vi "DataToSend.vi"(8 "error in (no error)":errorcluster, 9 "TimeStamp":timestamp, 10 "Data":string, 11 "Refnum":u64) -> (0 "error out":errorcluster, 3 "DataToSend":refnum<class "DataToSend.lvclass">)   [LabVIEW 2022 SP3, in "TcpServer.lvlib" / "DataToSend.lvclass"]
uses:
  DataToSend.lvclass
  DataToSend.lvclass/DataToSend.ctl
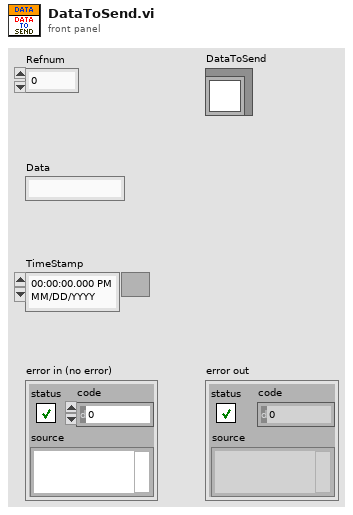
[diagram p1: front panel]
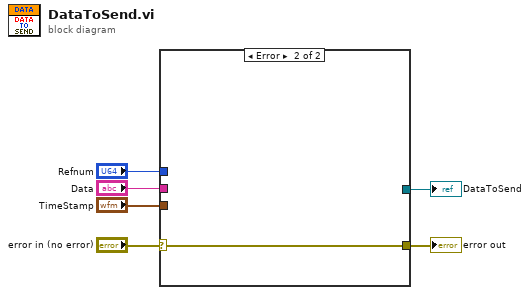
[diagram p0: block diagram]
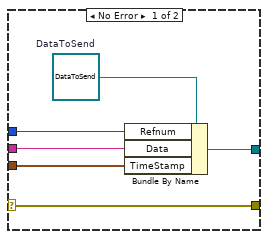
[diagram p2: hidden frame]
diagram:
  n1 = case shown="Error" "error in (no error)" {
    selector: "error in (no error)" -> [w12 w13]
    tunnel: [w12 w13] -> w5
    tunnel: [w10 _] -> w4
    tunnel: "TimeStamp" -> [w9 _]
    tunnel: "Data" -> [w8 _]
    tunnel: "Refnum" -> [w7 _]
    frame No Error {
      w11 = refnum<class "DataToSend.lvclass"> refnum  # DataToSend
      n2 = Bundle By Name(cluster=w11, "Refnum"=w7, "Data"=w8, "TimeStamp"=w9) -> (w10:refnum<class "DataToSend.lvclass">)
    }
    frame Error {
    }
  }
  "error out" <- w5
  "DataToSend" <- w4
